vi "Configure Overshoot.vi"(7 "Channel (0: Channel A)":u16(ring) items=["Channel A", "Channel B"], 8 "error in (no error)":errorcluster, 10 "Overshoot (1: Allowed)":u16(ring)=1 items=["Not Allowed", "Allowed"], 11 "BH Druck PACE Series in":refnum<class "BH Druck PACE Series.lvclass">) -> (0 "error out":errorcluster, 3 "BH Druck PACE Series out":refnum<class "BH Druck PACE Series.lvclass">)   [LabVIEW 2022 SP3, in "BH Druck PACE Series.lvclass"]
uses:
  BH Druck PACE Series.lvclass
  BH Druck PACE Series.lvclass/BH Druck PACE Series.ctl
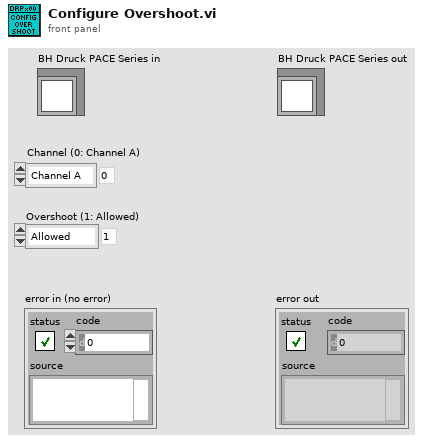
[diagram p1: front panel]
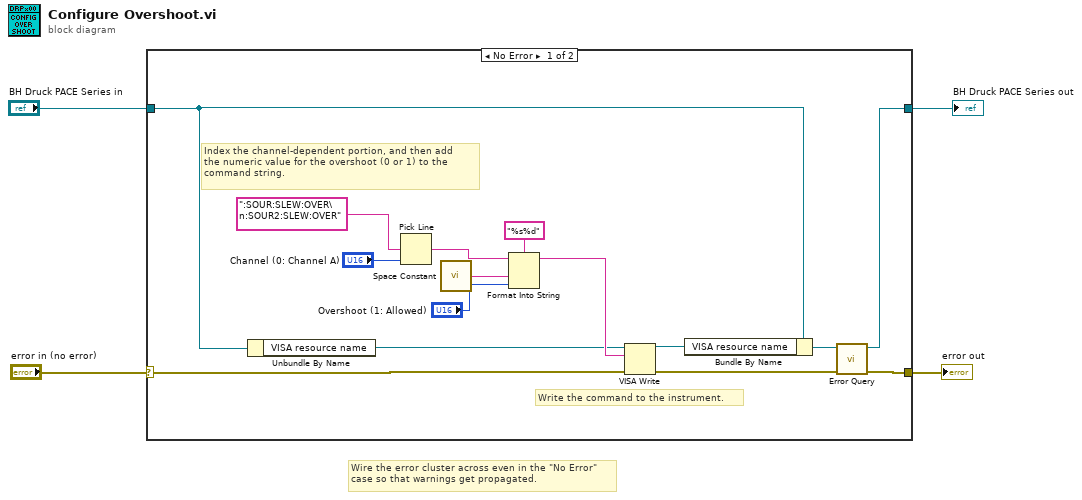
[diagram p0: block diagram]
diagram:
  # "Wire the error cluster across even in the \"No Error\"\ncase so that warnings get propagated."
  n1 = case shown="No Error" "error in (no error)" {
    selector: "error in (no error)" -> [w11 w21]
    tunnel: [w10 w21] -> w3
    tunnel: [w5 w20] -> w1
    tunnel: "BH Druck PACE Series in" -> [w8 w20]
    frame No Error {
      # "Index the channel-dependent portion, and then add\nthe numeric value for the overshoot (0 or 1) to the \ncommand string."
      # "Write the command to the instrument."
      n2 = Unbundle By Name(w8) -> ("VISA resource name"=w9:refnum<visa-resource-name>)
      n3 = Pick Line(multi-line string=":SOUR:SLEW:OVER\n:SOUR2:SLEW:OVER", line index="Channel (0: Channel A)") -> (output string=w15:string)  [unwired: 1 in]
      n4 = call <vilib>:"Space Constant.vi"() -> ("String"=w18:string)
      n5 = Format Into String(format string="%s%d", initial string=w15, w18, "Overshoot (1: Allowed)") -> (resulting string=w16:string)  [unwired: 1 in, 1 out]
      n6 = VISA Write(VISA resource name=w9, write buffer=w16, error in (no error)=w11) -> (VISA resource name out=w7:refnum<visa-resource-name>, error out=w19:errorcluster)  [unwired: 1 out]
      n7 = Bundle By Name(cluster=w8, "VISA resource name"=w7) -> (w6:refnum<class "BH Druck PACE Series.lvclass">)
      n8 = call-dynamic "Error Query.vi"("error in (no error)"=w19, "BH Druck PACE Series in"=w6) -> ("error out"=w10:errorcluster, "BH Druck PACE Series out"=w5:refnum<class "BH Druck PACE Series.lvclass">)  [unwired: 8 in]
    }
    frame Error {
    }
  }
  "error out" <- w3
  "BH Druck PACE Series out" <- w1
